vi "NATS Client request.vi"(6 "reply subject":string, 7 "timeout in ms (-1)":i32=-1, 8 "error in":errorcluster {"code" format="Error %.0f"}, 9 "payload":string, 10 "subject":string, 11 "NATS Client in":refnum<class "NATS Client.lvclass">) -> (0 "error out":errorcluster {"code" format="Error %.0f"}, 2 "time out":bool, 3 "nats message":T1)   [LabVIEW 2024, in "NATS Client.lvlib" / "NATS Client.lvclass"]
uses:
  NATS Client.lvclass
  Controls/nats message.ctl
  Controls/msg type.ctl
  NATS Client.lvclass/NATS Client.ctl
  VIs/NATS PUB.vi
  get nats connection.vi
  <vilib>/dlg_ctls.llb/Space Constant.vi
  VIs/subVIs/Set Timeout.vi
  NATS Subscription/NATS Subscription.lvclass
  NATS Core.lvlib
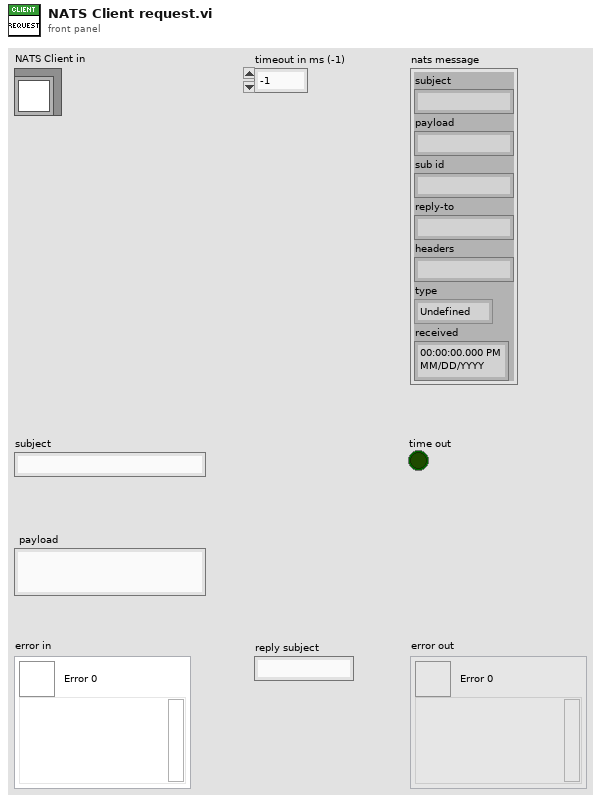
[diagram p1: front panel]
types:
  T1 = typedef "NATS Core.lvlib/nats message.ctl" = cluster{"subject":string, "payload":string, "sub id":string, "reply-to":string, "headers":string, "type":T2, "received":timestamp}
  T2 = typedef "NATS Core.lvlib/msg type.ctl" = enum16{"Undefined", "MSG", "HMSG", "+OK", "PING", "PONG", "-ERR", "INFO"}
  T3 = typedef "NATS Core.lvlib/nats connection.ctl" = cluster{"connection ID":refnum<k5>, "server INFO":string, "timeout ms":i32, "verbose?":bool, "server headers?":bool, "client headers?":bool}
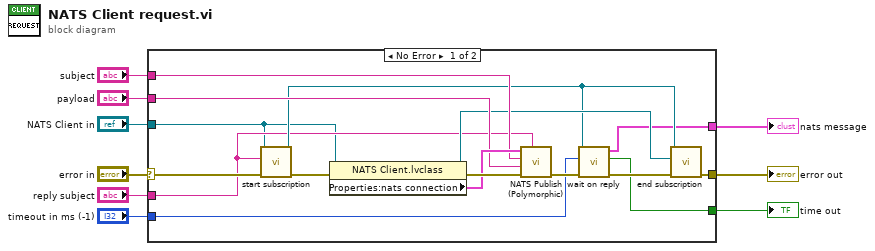
[diagram p0: block diagram]
diagram:
  n1 = case shown="No Error" "error in" {
    selector: "error in" -> [w22 w26]
    tunnel: [w23 w26] -> w8
    tunnel: "NATS Client in" -> [w13 _]
    tunnel: "payload" -> [w18 _]
    tunnel: "subject" -> [w17 _]
    tunnel: [w11 _] -> w4
    tunnel: "reply subject" -> [w14 _]
    tunnel: "timeout in ms (-1)" -> [w12 _]
    tunnel: [w10 _] -> w1
    frame No Error {
      n2 = call "start subscription.vi"("error in"=w22, "subject"=w14, "NATS Client"=w13) -> ("error out"=w21:errorcluster, "NATS Subscription"=w15:refnum<class "NATS Subscription.lvclass">)  [unwired: 7 in]
      n3 = property class="NATS Client.lvclass"(reference=w13, error in=w21) -> (reference out=w16:refnum<class "NATS Client.lvclass">, error out=w20:errorcluster, "Properties:nats connection"=w19:T3)
      n4 = call-poly "NATS Publish (Polymorphic).vi"("reply-to"=w14, "error in"=w20, "payload"=w18, "subject"=w17, "nats connection in"=w19) -> ("error out"=w25:errorcluster)  [unwired: 5 in, 1 out]
      n5 = call-dynamic "wait on reply.vi"("error in"=w25, "timeout in ms (-1)"=w12, "NATS Subscriber in"=w15) -> ("error out"=w24:errorcluster, "time out"=w10:bool, "nats message"=w11:T1)  [unwired: 6 in]
      n6 = call "end subscription.vi"("error in"=w24, "NATS Client"=w16, "NATS Subscription"=w15) -> ("error out"=w23:errorcluster)  [unwired: 8 in]
    }
    frame Error {
    }
  }
  "error out" <- w8
  "nats message" <- w4
  "time out" <- w1
